vi "Get Camera Information.vi"(10 "information":i32, 11 "index":i32) -> (2 "information out":i32, 3 "function return":u32)   [LabVIEW 2018, in "Copy of Andor SDK.lvlib"]
doc: "EXPNETTYPE unsigned int WINAPI GetCameraInformation(int index, long * information);"
uses:
  Copy of Andor SDK.lvlib
  <userlib>/Andor SDK/ATMCD32D.dll
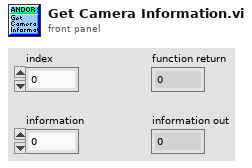
[diagram p1: front panel]
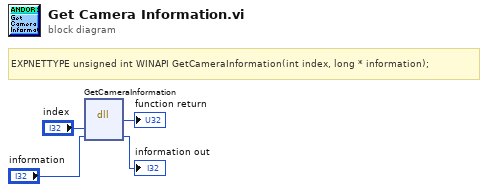
[diagram p0: block diagram]
diagram:
  # "EXPNETTYPE unsigned int WINAPI GetCameraInformation(int index, long * information);"
  n1 = dll-call lib="C:/Program Files (x86)/National Instruments/LabVIEW 2018/user.lib/Andor SDK/ATMCD32D.*" fn="GetCameraInformation"("index"="index", "information"="information") -> (→"function return":u32, "information"=→"information out":i32)  [unwired: 4 in, 2 out]
